vi "Treatment ROI.vi"(8 "error in (no error)":errorcluster, 10 "Treatment":T3, 11 "Limbus":T2) -> (0 "error out":errorcluster, 3 "ROI Descriptor":T1 {"Contours"."Type" items=["No Selection", "Point", "Line", "Rectangle", "Oval", "Polygon", "Freehand Region", "Annulus", "Unused2", "Unused3", "Broken Line", "Freehand Line", "Rotated Rectangle"]})   [LabVIEW 2015]
uses:
  controls/Treatment Parameters.ctl
  controls/Results.ctl
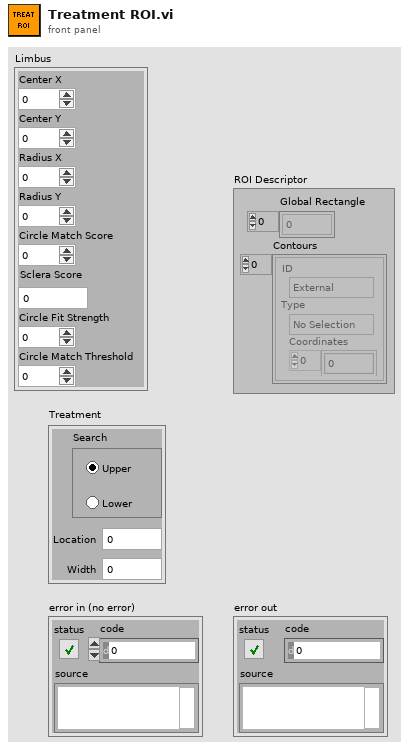
[diagram p1: front panel]
types:
  T1 = typedef "ROI Descriptor" = cluster{"Global Rectangle":i32[], "Contours":cluster{"ID":enum32{"External", "Internal"}, "Type":u32, "Coordinates":i32[]}[]}
  T2 = typedef "Results.ctl" = cluster{"Center X":i32, "Center Y":i32, "Radius X":i32, "Radius Y":i32, "Circle Match Score":i32, "Sclera Score":dbl, "Circle Fit Strength":i32, "Circle Match Threshold":i32}
  T3 = typedef "Treatment Parameters.ctl" = cluster{"Location":dbl, "Width":dbl, "Search":enum32{"Upper", "Lower"}}
  T4 = typedef "IMAQ Circle" = cluster{"Center X":i32, "Center Y":i32, "Inner Radius":i32, "Outer Radius":i32, "Start Angle":dbl, "End Angle":dbl}
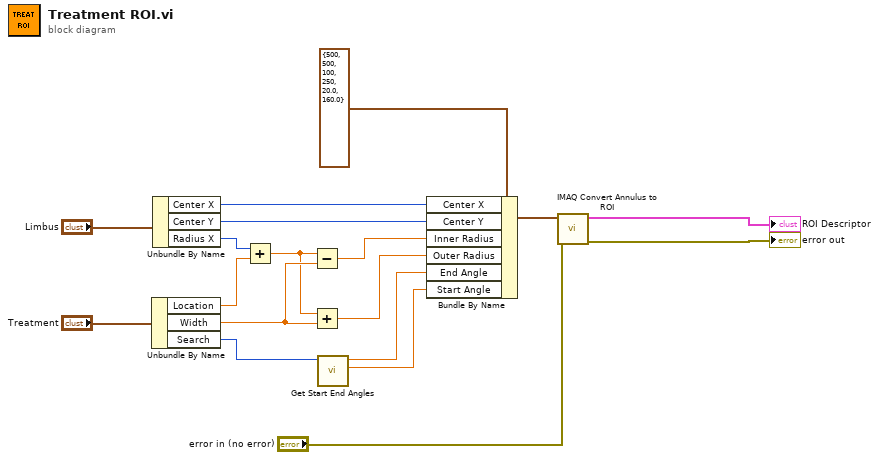
[diagram p0: block diagram]
diagram:
  n1 = Unbundle By Name("Treatment") -> ("Location"=w10:dbl, "Width"=w13:dbl, "Search"=w17:enum32{"Upper", "Lower"})
  n2 = Unbundle By Name("Limbus") -> ("Center X"=w6:i32, "Center Y"=w7:i32, "Radius X"=w8:i32)
  n3 = Add(x=w8, y=w10) -> (x+y=w12:dbl)
  n4 = Subtract(x=w12, y=w13) -> (x-y=w11:dbl)
  n5 = Add(x=w12, y=w13) -> (x+y=w14:dbl)
  n6 = call "Get Start End Angles.vi"("Search"=w17) -> ("Start Angle (degrees)"=w16:dbl, "End Angle (degrees)"=w15:dbl)  [unwired: 9 in]
  n7 = Bundle By Name(cluster=T4 {"Center X"=500, "Center Y"=500, "Inner Radius"=100, "Outer Radius"=250, "Start Angle"=20.0, "End Angle"=160.0} ("Annulus"), "Center X"=w6, "Center Y"=w7, "Inner Radius"=w11, "Outer Radius"=w14, "End Angle"=w15, "Start Angle"=w16) -> (w4:T4)
  n8 = call "IMAQ Convert Annulus to ROI"("error in (no error)"="error in (no error)", "Annulus"=w4) -> ("error out"=→"error out":errorcluster, "ROI Descriptor"=→"ROI Descriptor":T1)  [unwired: 7 in]
